vi "writefile.vi"(5 "Path":path, 6 "Save&Continue":bool, 7 "Save&Finish":bool, 8 "Polarity":i8, 9 "Sample Rate":i32=1000, 10 "Array":i16[][](array[numeric])) -> (2 "Path Out":path, 3 "Enum":T1)   [LabVIEW 2013]
uses:
  Lab/Undergraduates/Sarah_Sam/To Github/eodrecorderstates.ctl
panel:
  in  "Gain":i32
  in  "Coupling":bool
  in  "Temp":string="25"
  in  "Comments":string="Default values"
  in  "Species":string="Bennetti"
  in  "Location":string="EFish Lab"
  in  "Specimen":string="1"
  in  "Date":string="06/09/14"
  in  "Time":string="12:00:00"
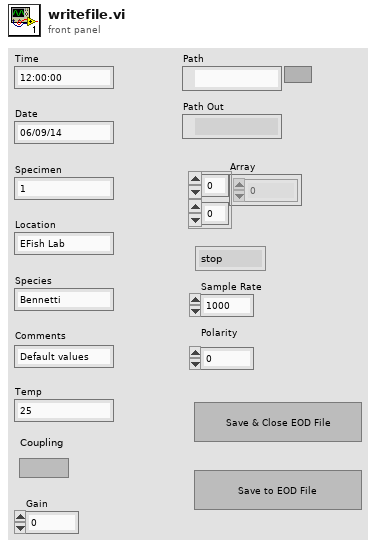
[diagram p1: front panel]
types:
  T1 = typedef "eodrecorderstates.ctl" = enum16{"stop", "initialize", "live data", "capture data", "analyze data", "open data", "display opened data", "write to file"}
  T2 = enum16{"big-endian, network order", "native, host order", "little-endian"}
  T3 = enum16{"open", "replace", "create", "open or create", "replace or create", "replace or create with confirmation"}
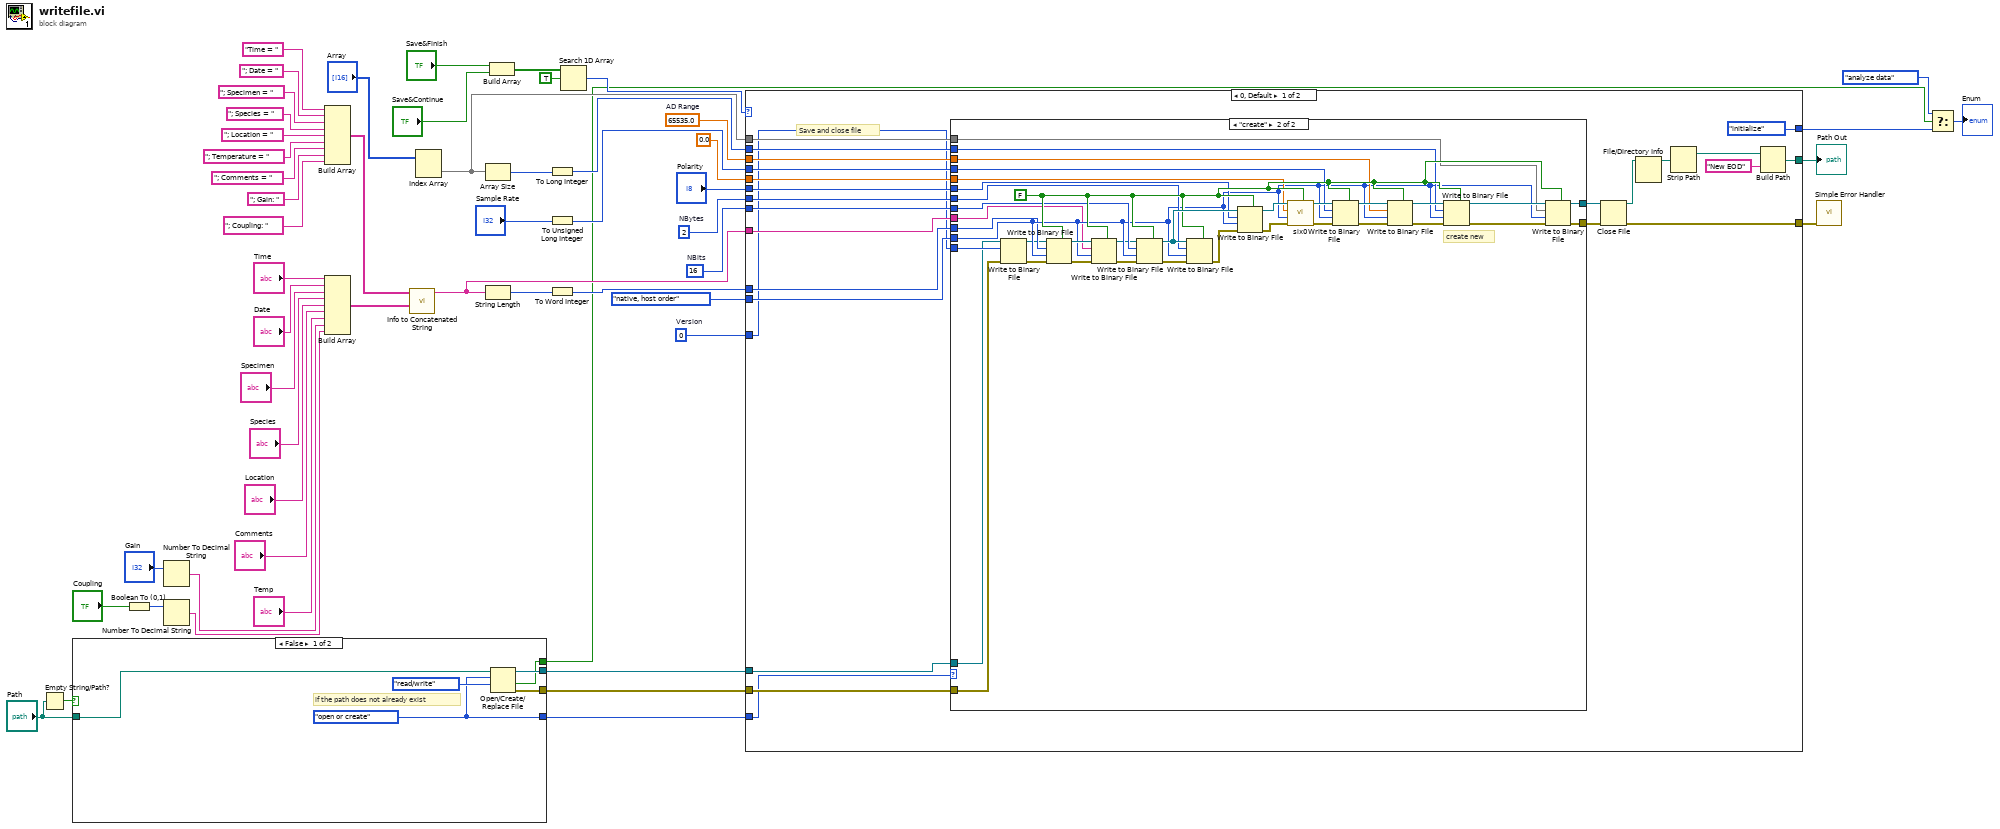
[diagram p0: block diagram]
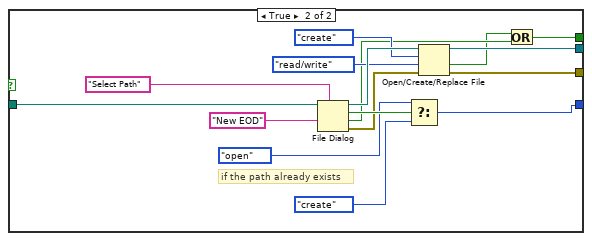
[diagram p2: hidden frame]
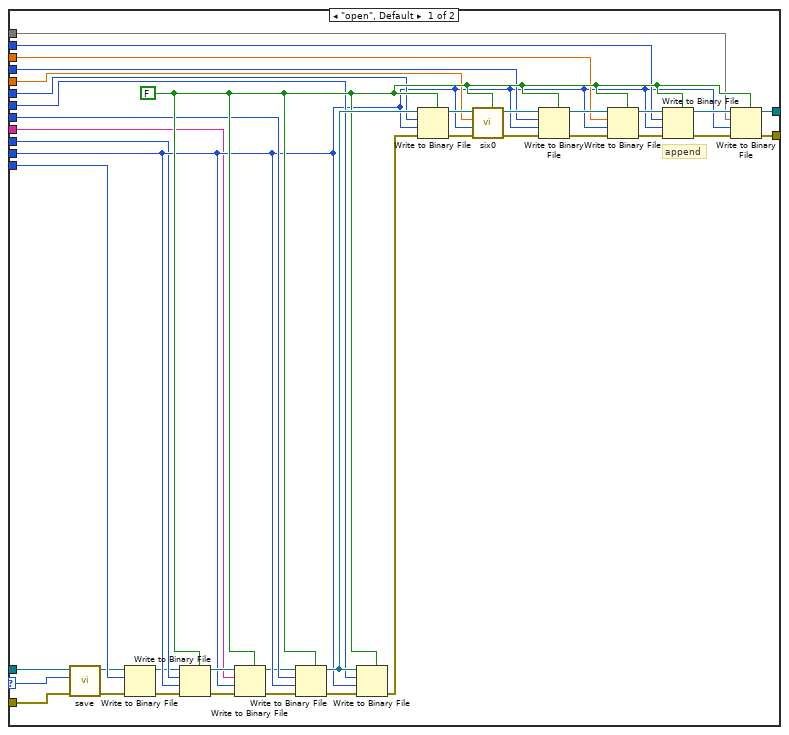
[diagram p3: hidden frame]
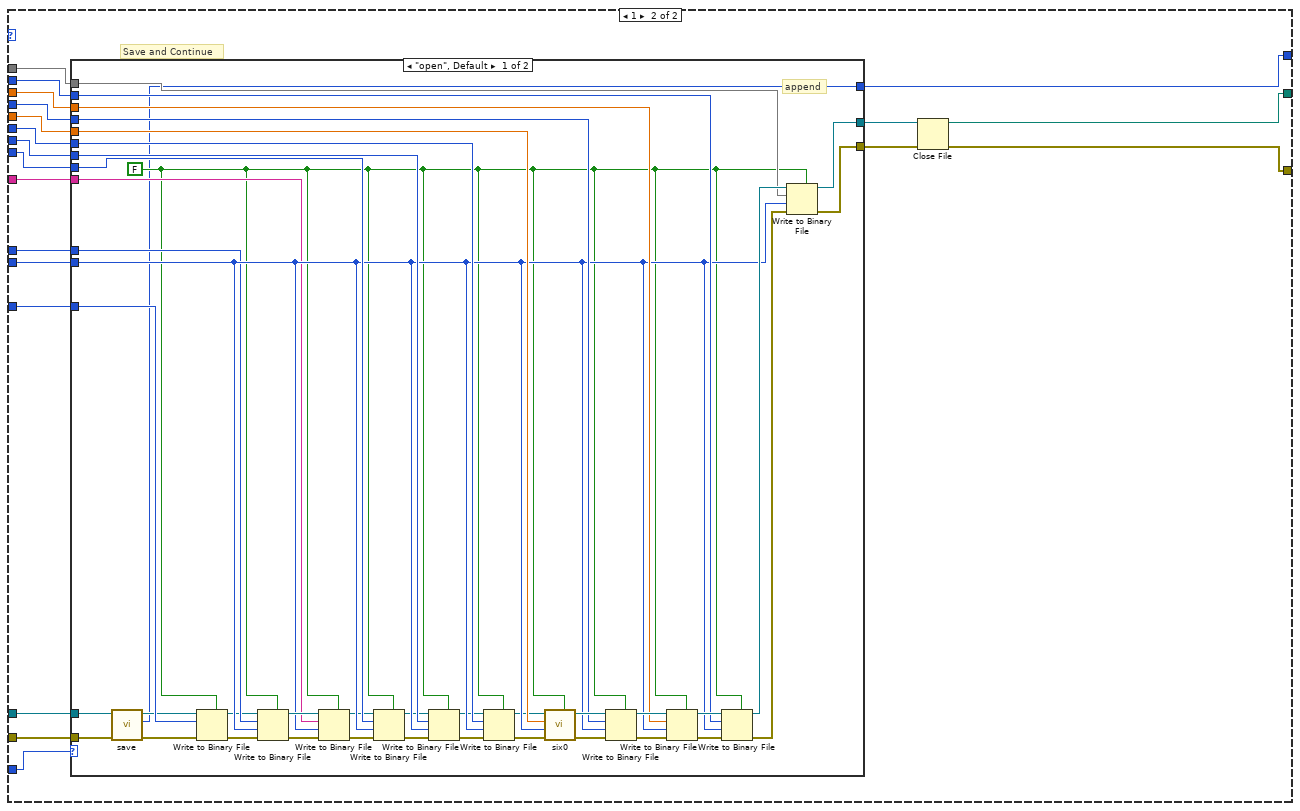
[diagram p4: hidden frame]
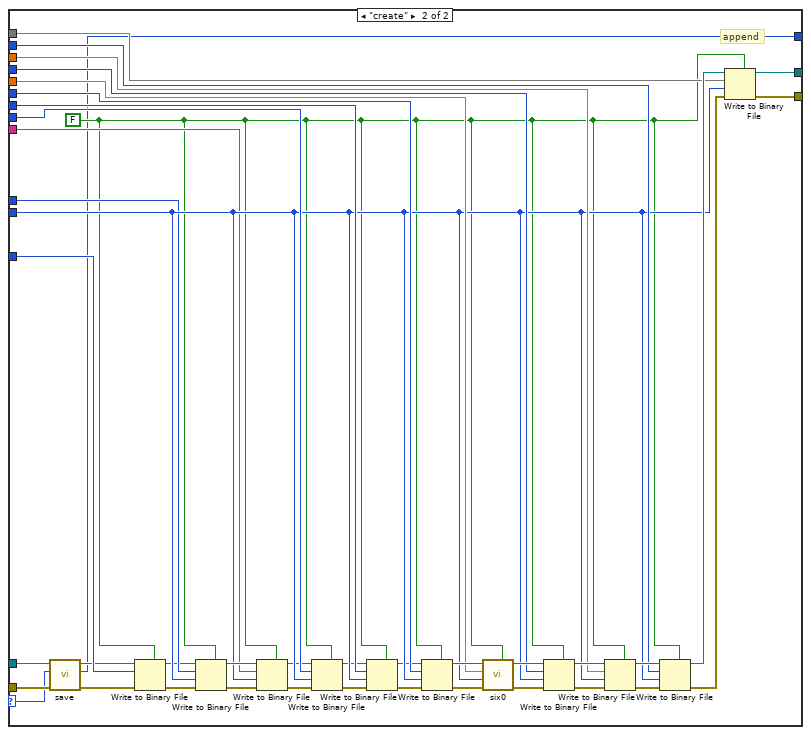
[diagram p5: hidden frame]
diagram:
  w33 = i8 2  # NBytes
  w37 = i8 0  # Version
  w30 = sgl 65535.0  # AD Range
  w34 = i8 16  # NBits
  n1 = Empty String/Path?(string/path="Path") -> (empty?=w15:bool)
  n2 = case shown="False" w15 {
    tunnel: "Path" -> [w60 w68]
    tunnel: [w59 w71] -> w18
    tunnel: [w58 w70] -> w20
    tunnel: [w57 w73] -> w19
    tunnel: [w56 w63] -> w10
    frame False {
      w57 = T3."open or create" ("operation (0:open)")
      # "if the path does not already exist"
      n3 = Open/Create/Replace File(file path (use dialog)=w60, operation (0:open)=w57, access (0:read/write)=enum16{"read/write", "read-only", "write-only"}."read/write") -> (refnum out=w59:refnum<file>, cancelled=w56:bool, error out=w58:errorcluster)  [unwired: 3 in]
    }
    frame True {
      # "if the path already exists"
      n4 = File Dialog(7:"Select Path", 9:"New EOD", 11:w68) -> (0:w69:errorcluster, 1:w64:bool, 2:w76:bool, 3:w72:path)  [unwired: 4 in]
      n5 = Select(t=T3."open" ("operation (0:open)"), s=w76, f=T3."create" ("operation (0:open)")) -> (s? t:f=w73:T3)
      n6 = Open/Create/Replace File(file path (use dialog)=w72, error in=w69, operation (0:open)=T3."create", access (0:read/write)=enum16{"read/write", "read-only", "write-only"}."read/write") -> (refnum out=w71:refnum<file>, cancelled=w62:bool, error out=w70:errorcluster)  [unwired: 2 in]
      n7 = Or(x=w62, y=w64) -> (x .or. y?=w63:bool)
    }
  }
  n8 = Boolean To (0,1)(Boolean="Coupling") -> (0, 1=w23:i16)
  n9 = Number To Decimal String(number="Gain") -> (decimal integer string=w21:string)  [unwired: 1 in]
  n10 = Number To Decimal String(number=w23) -> (decimal integer string=w22:string)  [unwired: 1 in]
  n11 = Build Array("Time = ", "; Date = ", "; Specimen = ", "; Species = ", "; Location = ", "; Temperature = ", "; Comments = ", "; Gain: ", "; Coupling: ") -> (w43:string[])
  n12 = Build Array("Time", "Date", "Specimen", "Species", "Location", "Comments", "Temp", w21, w22) -> (w44:string[])
  n13 = call "Info to Concatenated String.vi"("Info Array"=w44, "Title Array"=w43) -> ("Concatenated\nData"=w35:string)  [unwired: 9 in]
  n14 = Index Array(array="Array") -> (element=w27:i16[])  [unwired: 2 in]
  n15 = Array Size(array=w27) -> (size(s)=w41:i32)
  n16 = String Length(string=w35) -> (length=w42:i32)
  n17 = Build Array("Save&Finish", "Save&Continue") -> (w55:bool[])
  n18 = To Long Integer(number=w41) -> (32bit integer=w29:i32)
  n19 = To Unsigned Long Integer(number="Sample Rate") -> (unsigned 32bit integer=w32:u32)
  n20 = To Word Integer(number=w42) -> (16bit integer=w36:i16)
  n21 = Search 1D Array(1D array=w55, element=TRUE) -> (index of element=w14:i32)  [unwired: 1 in]
  n22 = case shown="0, Default" w14 {
    tunnel: [eodrecorderstates."initialize" w180] -> w13
    tunnel: w20 -> [w100 w196]
    tunnel: w18 -> [w99 w195]
    tunnel: T2."native, host order" ("byte order (0:big-endian, network order)") -> [w98 w194]
    tunnel: [w97 w193] -> w39
    tunnel: w36 -> [w95 w191]
    tunnel: w35 -> [w94 w190]
    tunnel: w34 -> [w93 w189]
    tunnel: w33 -> [w92 w188]
    tunnel: "Polarity" -> [w91 w187]
    tunnel: sgl 0.0 -> [w90 w186]
    tunnel: w32 -> [w89 w185]
    tunnel: w30 -> [w88 w184]
    tunnel: w29 -> [w87 w183]
    tunnel: w27 -> [w86 w182]
    tunnel: w37 -> [w85 w181]
    tunnel: w19 -> [w84 w179]
    tunnel: [w79 w177] -> w17
    frame 0, Default {
      # "Save and close file"
      n23 = case shown="\"create\"" w84 {
        selector: w84 -> [w102 _]
        tunnel: w100 -> [w113 w141]
        tunnel: w99 -> [w103 w142]
        tunnel: w98 -> [w116 w152]
        tunnel: [w111 w148] -> w96
        tunnel: [w112 w149] -> w83
        tunnel: w95 -> [w114 w150]
        tunnel: w94 -> [w115 w151]
        tunnel: w93 -> [w117 w153]
        tunnel: w92 -> [w124 w160]
        tunnel: w91 -> [w118 w154]
        tunnel: w90 -> [w119 w155]
        tunnel: w89 -> [w120 w156]
        tunnel: w88 -> [w121 w157]
        tunnel: w87 -> [w122 w158]
        tunnel: w86 -> [w123 w159]
        tunnel: w85 -> [w108 w146]
        frame "open", Default {
          w125 = FALSE ("prepend array or string size? (T)")
          # "append"
          n24 = call "save.vi"("error in (no error)"=w113, "operation"=w102, "Refnum in"=w103) -> ("error out"=w110:errorcluster, "Refnum out"=w107:refnum<file>)  [unwired: 6 in, 1 out]
          n25 = Write to Binary File(file (use dialog)=w107, data=w108, error in=w110) -> (refnum out=w106:refnum<file>, error out=w109:errorcluster)  [unwired: 3 in, 1 out]
          n26 = Write to Binary File(file (use dialog)=w106, data=w114, error in=w109, 5:w125, 9:w116) -> (refnum out=w140:refnum<file>, error out=w139:errorcluster)  [unwired: 1 in, 1 out]
          n27 = Write to Binary File(file (use dialog)=w140, data=w115, error in=w139, 5:w125, 9:w116) -> (refnum out=w105:refnum<file>, error out=w104:errorcluster)  [unwired: 1 in, 1 out]
          n28 = Write to Binary File(file (use dialog)=w105, data=w117, error in=w104, 5:w125, 9:w116) -> (refnum out=w138:refnum<file>, error out=w137:errorcluster)  [unwired: 1 in, 1 out]
          n29 = Write to Binary File(file (use dialog)=w138, data=w124, error in=w137, 5:w125, 9:w116) -> (error out=w136:errorcluster)  [unwired: 1 in, 2 out]
          n30 = Write to Binary File(file (use dialog)=w138, data=w118, error in=w136, 5:w125, 9:w116) -> (refnum out=w135:refnum<file>, error out=w134:errorcluster)  [unwired: 1 in, 1 out]
          n31 = call "six0.vi"("Boolean"=w125, "error in (no error)"=w134, "byte order (0:big-endian, network order)"=w116, "Numeric"=w119, "Byte Stream File in"=w135) -> ("error out"=w132:errorcluster, "Byte Stream File out"=w133:refnum<file>)  [unwired: 5 in]
          n32 = Write to Binary File(file (use dialog)=w133, data=w120, error in=w132, 5:w125, 9:w116) -> (refnum out=w131:refnum<file>, error out=w130:errorcluster)  [unwired: 1 in, 1 out]
          n33 = Write to Binary File(file (use dialog)=w131, data=w121, error in=w130, 5:w125, 9:w116) -> (refnum out=w129:refnum<file>, error out=w128:errorcluster)  [unwired: 1 in, 1 out]
          n34 = Write to Binary File(file (use dialog)=w129, data=w122, error in=w128, 5:w125, 9:w116) -> (refnum out=w127:refnum<file>, error out=w126:errorcluster)  [unwired: 1 in, 1 out]
          n35 = Write to Binary File(file (use dialog)=w127, data=w123, error in=w126, 5:w125, 9:w116) -> (refnum out=w112:refnum<file>, error out=w111:errorcluster)  [unwired: 1 in, 1 out]
        }
        frame "create" {
          w161 = FALSE ("prepend array or string size? (T)")
          # "create new"
          n36 = Write to Binary File(file (use dialog)=w142, data=w146, error in=w141) -> (refnum out=w145:refnum<file>, error out=w147:errorcluster)  [unwired: 3 in, 1 out]
          n37 = Write to Binary File(file (use dialog)=w145, data=w150, error in=w147, 5:w161, 9:w152) -> (refnum out=w176:refnum<file>, error out=w175:errorcluster)  [unwired: 1 in, 1 out]
          n38 = Write to Binary File(file (use dialog)=w176, data=w151, error in=w175, 5:w161, 9:w152) -> (refnum out=w143:refnum<file>, error out=w144:errorcluster)  [unwired: 1 in, 1 out]
          n39 = Write to Binary File(file (use dialog)=w143, data=w153, error in=w144, 5:w161, 9:w152) -> (refnum out=w174:refnum<file>, error out=w173:errorcluster)  [unwired: 1 in, 1 out]
          n40 = Write to Binary File(file (use dialog)=w174, data=w160, error in=w173, 5:w161, 9:w152) -> (error out=w172:errorcluster)  [unwired: 1 in, 2 out]
          n41 = Write to Binary File(file (use dialog)=w174, data=w154, error in=w172, 5:w161, 9:w152) -> (refnum out=w171:refnum<file>, error out=w170:errorcluster)  [unwired: 1 in, 1 out]
          n42 = call "six0.vi"("Boolean"=w161, "error in (no error)"=w170, "byte order (0:big-endian, network order)"=w152, "Numeric"=w155, "Byte Stream File in"=w171) -> ("error out"=w168:errorcluster, "Byte Stream File out"=w169:refnum<file>)  [unwired: 5 in]
          n43 = Write to Binary File(file (use dialog)=w169, data=w156, error in=w168, 5:w161, 9:w152) -> (refnum out=w167:refnum<file>, error out=w166:errorcluster)  [unwired: 1 in, 1 out]
          n44 = Write to Binary File(file (use dialog)=w167, data=w157, error in=w166, 5:w161, 9:w152) -> (refnum out=w165:refnum<file>, error out=w164:errorcluster)  [unwired: 1 in, 1 out]
          n45 = Write to Binary File(file (use dialog)=w165, data=w158, error in=w164, 5:w161, 9:w152) -> (refnum out=w163:refnum<file>, error out=w162:errorcluster)  [unwired: 1 in, 1 out]
          n46 = Write to Binary File(file (use dialog)=w163, data=w159, error in=w162, 5:w161, 9:w152) -> (refnum out=w149:refnum<file>, error out=w148:errorcluster)  [unwired: 1 in, 1 out]
        }
      }
      n47 = Close File(refnum=w83, error in=w96) -> (path=w81:path, error out=w97:errorcluster)
      n48 = File/Directory Info(path=w81) -> (path out=w82:path)  [unwired: 1 in, 6 out]
      n49 = Strip Path(path=w82) -> (stripped path=w80:path)  [unwired: 1 out]
      n50 = Build Path(base path=w80, name or relative path="New EOD") -> (appended path=w79:path)
    }
    frame 1 {
      # "Save and Continue"
      n51 = case shown="\"open\", Default" w179 {
        selector: w179 -> [_ w237]
        tunnel: w196 -> [w199 w242]
        tunnel: w195 -> [w197 w238]
        tunnel: w194 -> [w215 w255]
        tunnel: [w211 w251] -> w192
        tunnel: [w212 w252] -> w178
        tunnel: w191 -> [w213 w253]
        tunnel: w190 -> [w214 w254]
        tunnel: w189 -> [w216 w256]
        tunnel: w188 -> [w223 w263]
        tunnel: w187 -> [w217 w257]
        tunnel: w186 -> [w218 w258]
        tunnel: w185 -> [w219 w259]
        tunnel: w184 -> [w220 w260]
        tunnel: w183 -> [w221 w261]
        tunnel: w182 -> [w222 w262]
        tunnel: w181 -> [w205 w245]
        tunnel: [w198 w239] -> w180
        frame "open", Default {
          w206 = FALSE ("prepend array or string size? (T)")
          # "append"
          n52 = call "save.vi"("error in (no error)"=w199, "Refnum in"=w197) -> ("error out"=w200:errorcluster, "Recorder State"=w198:T1, "Refnum out"=w201:refnum<file>)  [unwired: 7 in]
          n53 = Write to Binary File(file (use dialog)=w201, data=w205, error in=w200, 5:w206) -> (refnum out=w207:refnum<file>, error out=w208:errorcluster)  [unwired: 2 in, 1 out]
          n54 = Write to Binary File(file (use dialog)=w207, data=w213, error in=w208, 5:w206, 9:w215) -> (refnum out=w236:refnum<file>, error out=w235:errorcluster)  [unwired: 1 in, 1 out]
          n55 = Write to Binary File(file (use dialog)=w236, data=w214, error in=w235, 5:w206, 9:w215) -> (refnum out=w204:refnum<file>, error out=w203:errorcluster)  [unwired: 1 in, 1 out]
          n56 = Write to Binary File(file (use dialog)=w204, data=w216, error in=w203, 5:w206, 9:w215) -> (refnum out=w210:refnum<file>, error out=w234:errorcluster)  [unwired: 1 in, 1 out]
          n57 = Write to Binary File(file (use dialog)=w210, data=w223, error in=w234, 5:w206, 9:w215) -> (refnum out=w209:refnum<file>, error out=w233:errorcluster)  [unwired: 1 in, 1 out]
          n58 = Write to Binary File(file (use dialog)=w209, data=w217, error in=w233, 5:w206, 9:w215) -> (refnum out=w202:refnum<file>, error out=w232:errorcluster)  [unwired: 1 in, 1 out]
          n59 = call "six0.vi"("Boolean"=w206, "error in (no error)"=w232, "byte order (0:big-endian, network order)"=w215, "Numeric"=w218, "Byte Stream File in"=w202) -> ("error out"=w230:errorcluster, "Byte Stream File out"=w231:refnum<file>)  [unwired: 5 in]
          n60 = Write to Binary File(file (use dialog)=w231, data=w219, error in=w230, 5:w206, 9:w215) -> (refnum out=w229:refnum<file>, error out=w228:errorcluster)  [unwired: 1 in, 1 out]
          n61 = Write to Binary File(file (use dialog)=w229, data=w220, error in=w228, 5:w206, 9:w215) -> (refnum out=w227:refnum<file>, error out=w226:errorcluster)  [unwired: 1 in, 1 out]
          n62 = Write to Binary File(file (use dialog)=w227, data=w221, error in=w226, 5:w206, 9:w215) -> (refnum out=w225:refnum<file>, error out=w224:errorcluster)  [unwired: 1 in, 1 out]
          n63 = Write to Binary File(file (use dialog)=w225, data=w222, error in=w224, 5:w206, 9:w215) -> (refnum out=w212:refnum<file>, error out=w211:errorcluster)  [unwired: 1 in, 1 out]
        }
        frame "create" {
          w246 = FALSE ("prepend array or string size? (T)")
          # "append"
          n64 = call "save.vi"("error in (no error)"=w242, "operation"=w237, "Refnum in"=w238) -> ("error out"=w241:errorcluster, "Recorder State"=w239:T1, "Refnum out"=w240:refnum<file>)  [unwired: 6 in]
          n65 = Write to Binary File(file (use dialog)=w240, data=w245, error in=w241, 5:w246) -> (refnum out=w247:refnum<file>, error out=w248:errorcluster)  [unwired: 2 in, 1 out]
          n66 = Write to Binary File(file (use dialog)=w247, data=w253, error in=w248, 5:w246, 9:w255) -> (refnum out=w277:refnum<file>, error out=w276:errorcluster)  [unwired: 1 in, 1 out]
          n67 = Write to Binary File(file (use dialog)=w277, data=w254, error in=w276, 5:w246, 9:w255) -> (refnum out=w244:refnum<file>, error out=w243:errorcluster)  [unwired: 1 in, 1 out]
          n68 = Write to Binary File(file (use dialog)=w244, data=w256, error in=w243, 5:w246, 9:w255) -> (refnum out=w250:refnum<file>, error out=w275:errorcluster)  [unwired: 1 in, 1 out]
          n69 = Write to Binary File(file (use dialog)=w250, data=w263, error in=w275, 5:w246, 9:w255) -> (refnum out=w249:refnum<file>, error out=w274:errorcluster)  [unwired: 1 in, 1 out]
          n70 = Write to Binary File(file (use dialog)=w249, data=w257, error in=w274, 5:w246, 9:w255) -> (refnum out=w273:refnum<file>, error out=w272:errorcluster)  [unwired: 1 in, 1 out]
          n71 = call "six0.vi"("Boolean"=w246, "error in (no error)"=w272, "byte order (0:big-endian, network order)"=w255, "Numeric"=w258, "Byte Stream File in"=w273) -> ("error out"=w270:errorcluster, "Byte Stream File out"=w271:refnum<file>)  [unwired: 5 in]
          n72 = Write to Binary File(file (use dialog)=w271, data=w259, error in=w270, 5:w246, 9:w255) -> (refnum out=w269:refnum<file>, error out=w268:errorcluster)  [unwired: 1 in, 1 out]
          n73 = Write to Binary File(file (use dialog)=w269, data=w260, error in=w268, 5:w246, 9:w255) -> (refnum out=w267:refnum<file>, error out=w266:errorcluster)  [unwired: 1 in, 1 out]
          n74 = Write to Binary File(file (use dialog)=w267, data=w261, error in=w266, 5:w246, 9:w255) -> (refnum out=w265:refnum<file>, error out=w264:errorcluster)  [unwired: 1 in, 1 out]
          n75 = Write to Binary File(file (use dialog)=w265, data=w262, error in=w264, 5:w246, 9:w255) -> (refnum out=w252:refnum<file>, error out=w251:errorcluster)  [unwired: 1 in, 1 out]
        }
      }
      n76 = Close File(refnum=w178, error in=w192) -> (path=w177:path, error out=w193:errorcluster)
    }
  }
  "Path Out" <- w17
  n77 = call <vilib>:"Simple Error Handler.vi"("error in (no error)"=w39) -> ()  [unwired: 4 in, 5 out]
  n78 = Select(t=eodrecorderstates."analyze data" ("Enum"), s=w10, f=w13) -> (s? t:f=→"Enum":T1)
